vi "Kmeans.vi"(9 "Point1":cluster{"X1":dbl, "Y1":dbl}, 10 "XYflipped":T1[](array[typedef]), 11 "3 random points in":T2={"Point1"={"X1"=150.0, "Y1"=150.0}, "Point2"={"X1"=300.0, "Y1"=300.0}, "Point3"={"X1"=0.0, "Y1"=0.0}}) -> (2 "VisualOut":cluster{dbl[], dbl[]}[](array[cluster])=[{[], []}, {[nan], [nan]}, {[nan], [nan]}, {[nan], [nan]}], 3 "3 random points out":T2={"Point1"={"X1"=nan, "Y1"=nan}, "Point2"={"X1"=nan, "Y1"=nan}, "Point3"={"X1"=nan, "Y1"=nan}})   [LabVIEW 2017]
uses:
  040-typeDefs/LidarPoint.ctl
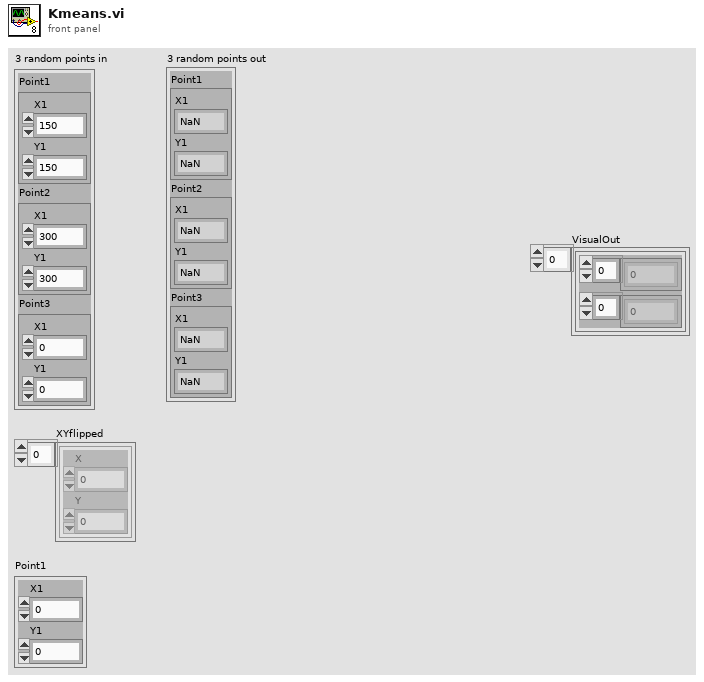
[diagram p1: front panel]
types:
  T1 = typedef "LidarPoint.ctl" = cluster{"X":dbl, "Y":dbl}
  T2 = cluster{"Point1":cluster{"X1":dbl, "Y1":dbl}, "Point2":cluster{"X1":dbl, "Y1":dbl}, "Point3":cluster{"X1":dbl, "Y1":dbl}}
  T3 = cluster{"Point1":cluster{"X1":bool, "Y1":bool}, "Point2":cluster{"X1":bool, "Y1":bool}, "Point3":cluster{"X1":bool, "Y1":bool}}
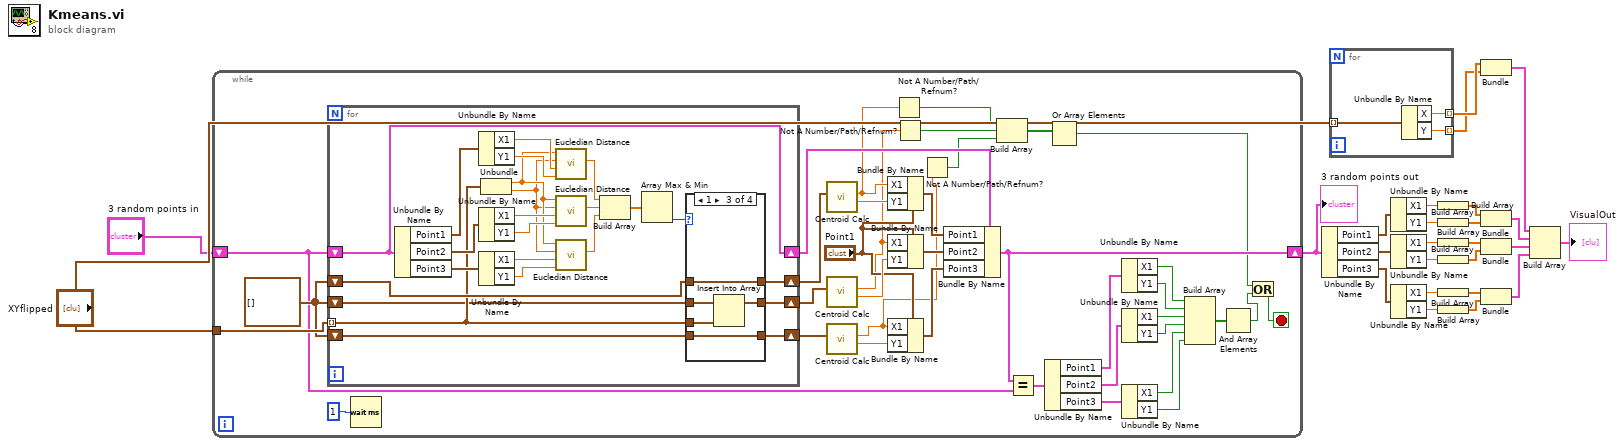
[diagram p0: block diagram]
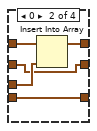
[diagram p3: hidden frame]
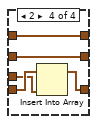
[diagram p4: hidden frame]
diagram:
  n1 = while {
    tunnel: "XYflipped" -> [w62]
    shift-right: [w49] -> w5
    shift-left: "3 random points in" -> [w48]
    stop <- w28 stop-if-true
    w61 = T1[] []
    n2 = for {
      tunnel: w62 -> [w69] mode=indexing
      shift-right: [w66] -> w60
      shift-left: w61 -> [w70]
      shift-right: [w67] -> w59
      shift-left: w61 -> [w68]
      shift-right: [w64] -> w58
      shift-left: w61 -> [w65]
      shift-right: [w63] -> w57
      shift-left: w48 -> [w63]
      n3 = Unbundle By Name(w63) -> ("Point1"=w86:cluster{"X1":dbl, "Y1":dbl}, "Point2"=w85:cluster{"X1":dbl, "Y1":dbl}, "Point3"=w84:cluster{"X1":dbl, "Y1":dbl})
      n4 = Unbundle By Name(w86) -> ("X1"=w83:dbl, "Y1"=w82:dbl)
      n5 = Unbundle By Name(w85) -> ("X1"=w81:dbl, "Y1"=w80:dbl)
      n6 = Unbundle By Name(w84) -> ("X1"=w77:dbl, "Y1"=w76:dbl)
      n7 = Unbundle(w69) -> ("X"=w79:dbl, "Y"=w78:dbl)
      n8 = call "Eucledian Distance.vi"("Y2"=w82, "X2"=w83, "Y"=w78, "X"=w79) -> ("Distance"=w75:dbl)  [unwired: 7 in]
      n9 = call "Eucledian Distance.vi"("Y2"=w80, "X2"=w81, "Y"=w78, "X"=w79) -> ("Distance"=w74:dbl)  [unwired: 7 in]
      n10 = call "Eucledian Distance.vi"("Y2"=w76, "X2"=w77, "Y"=w78, "X"=w79) -> ("Distance"=w73:dbl)  [unwired: 7 in]
      n11 = Build Array(w75, w74, w73) -> (w72:dbl[])
      n12 = Array Max & Min(array=w72) -> (min index (indices)=w71:i32)  [unwired: 3 out]
      n13 = case shown="1" w71 {
        tunnel: w70 -> [w89 w94 w96 w101]
        tunnel: w69 -> [_ w93 w98 w103]
        tunnel: w68 -> [w88 w91 w99 w100]
        tunnel: [w88 w91 w97 w100] -> w67
        tunnel: [w89 w92 w96 w101] -> w66
        tunnel: w65 -> [w87 w90 w95 w104]
        tunnel: [w87 w90 w95 w102] -> w64
        frame Default {
        }
        frame 0 {
          n14 = Insert Into Array(array=w94, new element=w93) -> (w92:T1[])  [unwired: 1 in]
        }
        frame 1 {
          n15 = Insert Into Array(array=w99, new element=w98) -> (w97:T1[])  [unwired: 1 in]
        }
        frame 2 {
          n16 = Insert Into Array(array=w104, new element=w103) -> (w102:T1[])  [unwired: 1 in]
        }
      }
    }
    n17 = Wait (ms)(milliseconds to wait=u32 1) -> ()  [unwired: 1 out]
    n18 = call "Centroid Calc.vi"("Array"=w60) -> ("Y Centroid"=w56:dbl, "X Centroid"=w35:dbl)  [unwired: 9 in]
    n19 = call "Centroid Calc.vi"("Array"=w59) -> ("Y Centroid"=w55:dbl, "X Centroid"=w34:dbl)  [unwired: 9 in]
    n20 = call "Centroid Calc.vi"("Array"=w58) -> ("Y Centroid"=w54:dbl, "X Centroid"=w33:dbl)  [unwired: 9 in]
    n21 = Bundle By Name(cluster="Point1", "X1"=w35, "Y1"=w56) -> (w53:cluster{"X1":dbl, "Y1":dbl})
    n22 = Bundle By Name(cluster="Point1", "X1"=w34, "Y1"=w55) -> (w52:cluster{"X1":dbl, "Y1":dbl})
    n23 = Bundle By Name(cluster="Point1", "X1"=w33, "Y1"=w54) -> (w51:cluster{"X1":dbl, "Y1":dbl})
    n24 = Not A Number/Path/Refnum?(number/path/refnum=w35) -> (NaN/Path/Refnum?=w32:bool)
    n25 = Not A Number/Path/Refnum?(number/path/refnum=w34) -> (NaN/Path/Refnum?=w31:bool)
    n26 = Not A Number/Path/Refnum?(number/path/refnum=w33) -> (NaN/Path/Refnum?=w30:bool)
    n27 = Bundle By Name(cluster=w57, "Point1"=w53, "Point2"=w52, "Point3"=w51) -> (w49:T2)
    n28 = Build Array(w32, w31, w30) -> (w29:bool[])
    n29 = Equal?(x=w49, y=w48) -> (x = y?=w47:T3)
    n30 = Unbundle By Name(w47) -> ("Point1"=w46:cluster{"X1":bool, "Y1":bool}, "Point2"=w45:cluster{"X1":bool, "Y1":bool}, "Point3"=w44:cluster{"X1":bool, "Y1":bool})
    n31 = Or Array Elements(Boolean array=w29) -> (logical OR=w26:bool)
    n32 = Unbundle By Name(w46) -> ("X1"=w43:bool, "Y1"=w42:bool)
    n33 = Unbundle By Name(w45) -> ("X1"=w41:bool, "Y1"=w40:bool)
    n34 = Unbundle By Name(w44) -> ("X1"=w39:bool, "Y1"=w38:bool)
    n35 = Build Array(w43, w42, w41, w40, w39, w38) -> (w37:bool[])
    n36 = And Array Elements(Boolean array=w37) -> (logical AND=w27:bool)
    n37 = Or(x=w26, y=w27) -> (x .or. y?=w28:bool)
  }
  "3 random points out" <- w5
  n38 = Unbundle By Name(w5) -> ("Point1"=w6:cluster{"X1":dbl, "Y1":dbl}, "Point2"=w7:cluster{"X1":dbl, "Y1":dbl}, "Point3"=w8:cluster{"X1":dbl, "Y1":dbl})
  n39 = for {
    tunnel: "XYflipped" -> [w107] mode=indexing
    tunnel: [w106] -> w3 mode=indexing
    tunnel: [w105] -> w2 mode=indexing
    n40 = Unbundle By Name(w107) -> ("X"=w106:dbl, "Y"=w105:dbl)
  }
  n41 = Unbundle By Name(w6) -> ("X1"=w9:dbl, "Y1"=w10:dbl)
  n42 = Unbundle By Name(w7) -> ("X1"=w11:dbl, "Y1"=w12:dbl)
  n43 = Unbundle By Name(w8) -> ("X1"=w13:dbl, "Y1"=w20:dbl)
  n44 = Build Array(w9) -> (w14:dbl[])
  n45 = Build Array(w10) -> (w15:dbl[])
  n46 = Build Array(w11) -> (w16:dbl[])
  n47 = Build Array(w12) -> (w17:dbl[])
  n48 = Build Array(w13) -> (w18:dbl[])
  n49 = Build Array(w20) -> (w19:dbl[])
  n50 = Bundle(w3, w2) -> (w24:cluster{dbl[], dbl[]})  [unwired: 1 in]
  n51 = Bundle(w14, w15) -> (w21:cluster{dbl[], dbl[]})  [unwired: 1 in]
  n52 = Bundle(w16, w17) -> (w22:cluster{dbl[], dbl[]})  [unwired: 1 in]
  n53 = Bundle(w18, w19) -> (w23:cluster{dbl[], dbl[]})  [unwired: 1 in]
  n54 = Build Array(w24, w21, w22, w23) -> (→"VisualOut":cluster{dbl[], dbl[]}[])
